vi "Report Freq Err.vi"(8 "error in (no error)":errorcluster, 11 "FreqErr":dbl) -> (0 "error out":errorcluster)   [LabVIEW 2013, in "QCAWLAN_DLL.lvlib"]
doc: "QCA_DLL_Export void ReportFreqErr(double FreqErr);"
uses:
  QCAWLAN_DLL.lvlib
  QCAWLAN_DLL.dll
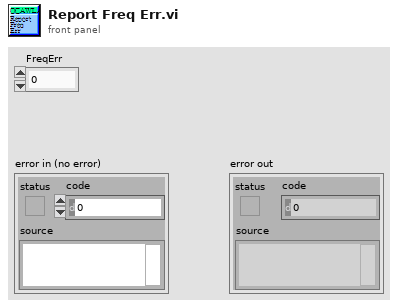
[diagram p1: front panel]
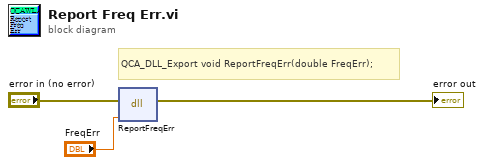
[diagram p0: block diagram]
diagram:
  # "QCA_DLL_Export void ReportFreqErr(double FreqErr);"
  n1 = dll-call lib="C:/Connectivity Client - MIMO/PlugIn/QCAWLAN_DLL.*" fn="ReportFreqErr"(error in="error in (no error)", "FreqErr"="FreqErr") -> (error out=→"error out":errorcluster)  [unwired: 4 in, 1 out]
